vi "VelocityFromPositionDerivative.vi"(10 "Control Loop Period [s]":dbl, 11 "Position [deg]":dbl) -> (3 "Velocity":dbl)   [LabVIEW 2019]
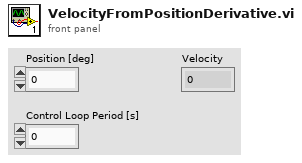
[diagram p1: front panel]
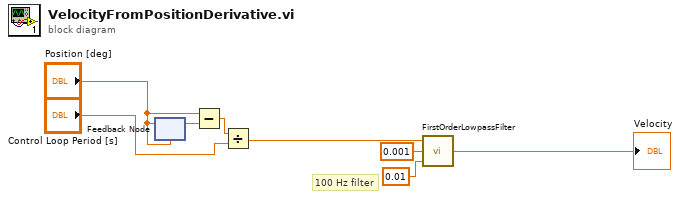
[diagram p0: block diagram]
diagram:
  # "100 Hz filter"
  n1 = feedback #1("Position [deg]") -> (w5:dbl)
  n2 = feedback-in #1("Position [deg]") -> ()
  n3 = Subtract(x="Position [deg]", y=w5) -> (x-y=w6:dbl)
  n4 = Divide(x=w6, y="Control Loop Period [s]") -> (x/y=w4:dbl)
  n5 = call "FirstOrderLowpassFilter.vi"("Tf"=0.01, "Ts"=0.001, "u"=w4) -> ("y"=→"Velocity":dbl)
